vi "HWIn Loop.vi"(11 "RT Data":T1 {"Label Transfer Config"."Block Data Refs"."Data Reference" format="%.0x"; "Status Config"."HWOut Dur Ref" format="%.0x"; "Status Config"."HWIn Dur Ref" format="%.0x"; "Status Config"."Error Data Ref" format="%.0x"; "HWOutput Channels"."Labels Settings"."Label" format="%.0o"; "HWInput Channels"."Labels Settings"."Label" format="%.0o"}) -> ()   [LabVIEW 2012, in "AIT 429 Engine.lvlib"]
uses:
  AIT 429 Engine.lvlib
  RT Controls/RT Data.ctl
  RT Controls/RT HW Channel.ctl
  RT Controls/RT Label Settings.ctl
  Shared/Controls and Global/Label.ctl
  Shared/Controls and Global/transferPeriod.ctl
  RT Controls/Driver Data.ctl
  RT Controls/RT Word Settings.ctl
  <vilib>/NI Veristand/Custom Device API/Block Data Reference.ctl
  <vilib>/NI Veristand/Custom Device API/Data Reference.ctl
  RT Controls/RT Param Setting.ctl
  Shared/Controls and Global/Start Bit.ctl
  Shared/Controls and Global/Number of Bits.ctl
  Shared/Controls and Global/TransferType.ctl
  RT Controls/Error Qs.ctl
  RT Controls/Status Channels Config.ctl
  RT Controls/FIFO.ctl
  RT Controls/Label Transfer Config.ctl
  SEA 9811 FPGA driver/RT/Typdefs/SEA9811_RT_data_cluster.ctl
  SEA 9811 FPGA driver/RT/Typdefs/FPGA ref.ctl
  SEA 9811 FPGA driver/RT/Typdefs/channel.ctl
  SEA 9811 FPGA driver/RT/Typdefs/received word.ctl
  <vilib>/Platform/TimedLoop/XDataNode/timing_clust.ctl
  <vilib>/Platform/TimedLoop/XDataNode/nitl_modes.ctl
  <vilib>/Platform/TimedLoop/XDataNode/wakeup.ctl
  RT Controls/ReadWrite Selector.ctl
  SubVIs/ReadWrite/Read FIFOs.vi
  SubVIs/ReadWrite/Write FIFOs.vi
  SubVIs/ReadWrite/ReadWrite TransConfig.vi
  SubVIs/ReadWrite/ReadWrite LoopStats.vi
  <vilib>/NI Veristand/Custom Device API/NI VeriStand - Get Channel Values by Block Data Reference.vi
  <vilib>/NI Veristand/Custom Device API/NI VeriStand - Set Channel Value by Data Reference.vi
  SubVIs/ReadWrite/ReadWrite All Data.vi
  <vilib>/Platform/TimedLoop/XDataNode/XDataNode.xnode
  <vilib>/Platform/TimedLoop/XDataNode/XDNodeRunTimeDep.lvlib
  Shared/ARINC 429 Shared.lvlib
  <vilib>/NI Veristand/Custom Device API/Custom Device API.lvlib
panel:
  in  "stop":bool
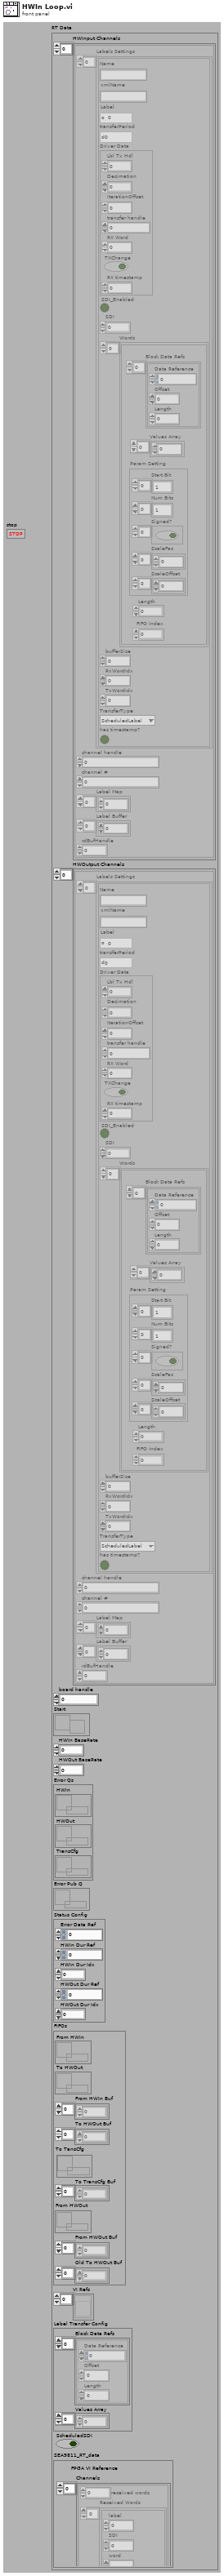
[diagram p1: front panel]
types:
  T1 = typedef "AIT 429 Engine.lvlib/RT Data.ctl" = cluster{"HWInput Channels":T2[], "HWOutput Channels":T2[], "board handle":u32, "Start":refnum<notifier>, "HWIn BaseRate":i64, "HWOut BaseRate":i64, "Error Qs":T14, "Error Pub Q":refnum<queue>, "Status Config":T15, "FIFOs":T16, "VI Refs":refnum<vi>[], "Label Transfer Config":T17, "ScheduledSDI":bool, "SEA9811_RT_data":T18}
  T2 = typedef "AIT 429 Engine.lvlib/RT HW Channel.ctl" = cluster{"Labels Settings":T3[], "channel handle":u32, "channel #":u16, "Label Map":i32[], "Label Buffer":u32[], "rdBufHandle":u32}
  T3 = typedef "AIT 429 Engine.lvlib/RT Label Settings.ctl" = cluster{"Name":string, "xmlName":string, "Label":T4, "transferPeriod":T5, "Driver Data":T6, "SDI_Enabled":bool, "SDI":u8, "Words":T7[], "bufferSize":u32, "RxWordIdx":i32, "TxWordIdx":i32, "TransferType":T13, "has timestamp?":bool}
  T4 = typedef "ARINC 429 Shared.lvlib/Label.ctl" = u8
  T5 = typedef "ARINC 429 Shared.lvlib/transferPeriod.ctl" = u32
  T6 = typedef "AIT 429 Engine.lvlib/Driver Data.ctl" = cluster{"Lbl Tx Hdl":u32, "Decimation":i32, "IterationOffset":i32, "transfer handle":u32, "RX Word":u32, "TXChange":bool, "RX timestamp":dbl}
  T7 = typedef "AIT 429 Engine.lvlib/RT Word Settings.ctl" = cluster{"Block Data Refs":T8[], "Values Array":dbl[], "Length":i32, "FIFO Index":i32, "Param Setting":T10}
  T8 = typedef "Custom Device API.lvlib/Block Data Reference.ctl" = cluster{"Data Reference":T9, "Offset":i32, "Length":i32}
  T9 = typedef "Custom Device API.lvlib/Data Reference.ctl" = i32
  T10 = typedef "AIT 429 Engine.lvlib/RT Param Setting.ctl" = cluster{"Start Bit":T11[], "Num Bits":T12[], "Signed?":bool[], "ScaleFac":dbl[], "ScaleOffset":dbl[]}
  T11 = typedef "ARINC 429 Shared.lvlib/Start Bit.ctl" = i32
  T12 = typedef "ARINC 429 Shared.lvlib/Number of Bits.ctl" = i32
  T13 = typedef "ARINC 429 Shared.lvlib/TransferType.ctl" = enum16{"ScheduledLabel", "Acyclic", "Block", "Strobe"}
  T14 = typedef "AIT 429 Engine.lvlib/Error Qs.ctl" = cluster{"HWIn":refnum<queue>, "HWOut":refnum<queue>, "TransCfg":refnum<queue>}
  T15 = typedef "AIT 429 Engine.lvlib/Status Channels Config.ctl" = cluster{"Error Data Ref":T9, "HWIn Dur Ref":T9, "HWIn Dur Idx":i32, "HWOut Dur Ref":T9, "HWOut Dur Idx":i32}
  T16 = typedef "AIT 429 Engine.lvlib/FIFO.ctl" = cluster{"From HWIn":refnum<k33>, "To HWOut":refnum<k33>, "From HWIn Buf":dbl[], "To HWOut Buf":dbl[], "To TansCfg":refnum<k33>, "To TransCfg Buf":dbl[], "From HWOut":refnum<k33>, "From HWOut Buf":dbl[], "Old To HWOut Buf":dbl[]}
  T17 = typedef "AIT 429 Engine.lvlib/Label Transfer Config.ctl" = cluster{"Block Data Refs":T8[], "Values Array":dbl[]}
  T18 = typedef "SEA9811_RT_data_cluster.ctl" = cluster{"FPGA VI Reference":T19, "Channels":T20[]}
  T19 = typedef "FPGA ref.ctl" = refnum<k20>
  T20 = typedef "channel.ctl" = cluster{"received words":u32, "Received Words":T21[]}
  T21 = typedef "received word.ctl" = cluster{"label":u8, "SDI":u8, "word":u32, "timestamp":dbl}
  T22 = typedef "AIT 429 Engine.lvlib/ReadWrite Selector.ctl" = enum16{"Inline Read", "Inline Write", "Async HWIn", "Async HWOut"}
  T23 = typedef "XDNodeRunTimeDep.lvlib/timing_clust.ctl" = cluster{"Expected End [f-1]":u64, "Actual End [f-1]":u64, "Finished Late? [f-1]":bool, "Expected End [i-1]":u64, "Actual End [i-1]":u64, "Finished Late? [i-1]":bool, "Expected Start [i]":u64, "Actual Start [i]":u64, "Expected Start [f]":u64, "Actual Start [f]":u64, "Source Name":string, "Structure Name":string, "Period":i64, "Deadline":i64, "Offset":i64, "Start":i64, "Priority":i32, "Timeout":i32, "Mode":T24, "Wakeup Reason":T25, "Error":errorcluster, "Source Type":string, "Secondary Source Type":string, "Global End Time":u64, "Global Start Time":u64, "Frame Duration":u64, "Iteration Duration":u64, "Assigned CPU":i32, "I/O Scan Engine Mode":u32}
  T24 = typedef "XDNodeRunTimeDep.lvlib/nitl_modes.ctl" = enum32{"No Change", "Process missed periods, maintain original phase", "Discard missed periods, maintain original phase", "Process missed periods, ignore original phase", "Discard missed periods, ignore original phase"}
  T25 = typedef "XDNodeRunTimeDep.lvlib/wakeup.ctl" = enum32{"Normal", "Aborted", "Asynchronous wakeup", "Timing source error", "Timed loop error", "Timeout"}
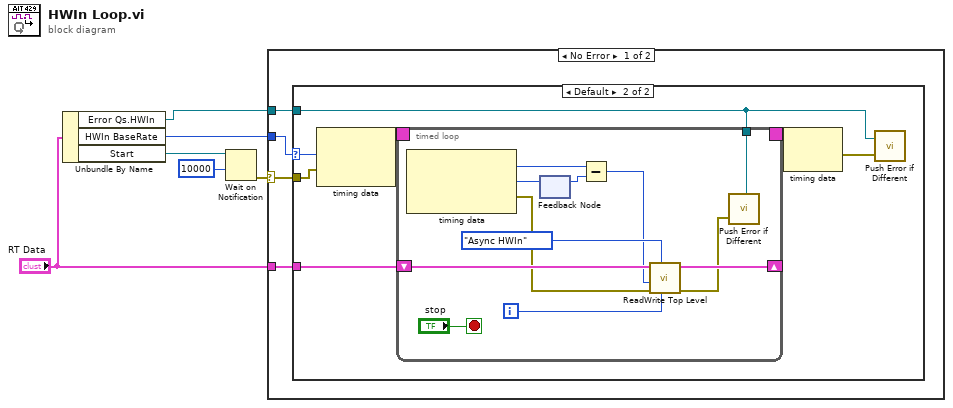
[diagram p0: block diagram]
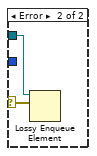
[diagram p3: hidden frame]
diagram:
  n1 = Unbundle By Name("RT Data") -> ("Error Qs.HWIn"=w1:refnum<queue>, "HWIn BaseRate"=w6:i64, "Start"=w5:refnum<notifier>)
  n2 = Wait on Notification(notifier=w5, timeout in ms (-1)=10000) -> (error out=w4:errorcluster)  [unwired: 2 in, 3 out]
  n3 = case shown="No Error" w4 {
    selector: w4 -> [w8 w42]
    tunnel: w6 -> [w7 _]
    tunnel: "RT Data" -> [w10 _]
    tunnel: w1 -> [w9 w41]
    frame No Error {
      n4 = case shown="Default" w7 {
        selector: w7 -> [_ w11]
        tunnel: w10 -> [_ w15]
        tunnel: w9 -> [_ w13]
        tunnel: w8 -> [_ w12]
        frame -1 {
        }
        frame Default {
          n5 = node-c288(w11, w12) -> (w17:T23)
          n6 = timed-loop {
            timing: w17 -> [_]
            timing-out: [_] -> w16
            shift-right: [w27] -> _
            shift-left: w15 -> [w28]
            tunnel: w13 -> [w24]
            i -> [w23]
            stop <- "stop" stop-if-true
            n7 = node-c288() -> (w20:i64, w22:i64, w18:errorcluster)  [unwired: 1 in]
            n8 = feedback-in #1(w22) -> ()
            n9 = feedback #1() -> (w21:i64)  [unwired: 1 in]
            n10 = Subtract(x=w20, y=w21) -> (x-y=w19:i64)
            n11 = call "ReadWrite Top Level.vi"("Iteration"=w23, "Mode"=ReadWrite_Selector."Async HWIn", "error in (no error)"=w18, "Iteration Duration"=w19, "RT Data in"=w28) -> ("error out"=w25:errorcluster, "RT Data out"=w27:T1)  [unwired: 5 in]
            n12 = call "Push Error if Different.vi"("error in"=w25, "Error Q"=w24) -> ()  [unwired: 1 in]
          }
          n13 = node-c288(w16) -> (w14:errorcluster)
          n14 = call "Push Error if Different.vi"("error in"=w14, "Error Q"=w13) -> ()  [unwired: 1 in]
        }
      }
    }
    frame Error {
      n15 = Lossy Enqueue Element(queue=w41, element=w42) -> ()  [unwired: 1 in, 4 out]
    }
  }
